vi "String is valid filename.vi"(4 "String":string) -> (1 "Is valid filename?":bool)   [LabVIEW 2011, in "COSYLib.lvlib"]
doc: "Checks if a string contains any characters that are invalid in a Windows filename, and if the string has at least length 1.\nNote that this is not a guarantee that the string is a valid filename, but it should take care of most common cases."
uses:
  COSYLib.lvlib
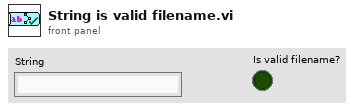
[diagram p1: front panel]
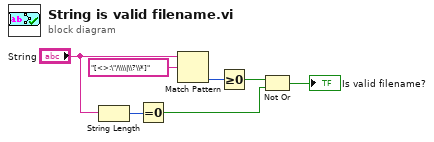
[diagram p0: block diagram]
diagram:
  n1 = String Length(string="String") -> (length=w3:i32)
  n2 = Equal To 0?(x=w3) -> (x = 0?=w1:bool)
  n3 = Match Pattern(string="String", regular expression="[<>:\"/\\\\|\\?\\*]") -> (offset past match=w6:i32)  [unwired: 1 in, 3 out]
  n4 = Greater Or Equal To 0?(x=w6) -> (x >= 0?=w5:bool)
  n5 = Not Or(1:w1, 2:w5) -> (0:→"Is valid filename?":bool)
